vi "InvFourierTransform.vi"(2 "Complex matrix":cdb[][](array[numeric]) format="%.2f", 3 "Image In":T1 {"Dialogs" format="%.0b"}) -> (1 "Image Out":T1 {"Dialogs" format="%.0b"})   [LabVIEW 2024]
doc: "This VI calculates the inverse DFT (or FFT) of the complex matrix and returns the resulting real the image. It only works on greyscale images."
uses:
  <userlib>/ImageProcessing/QTLIB_2595_LV86/QT_Image.ctl
panel:
  # "This VI calculates the inverse DFT (or FFT) of the complex matrix and returns the resulting real the image.  It only works on greyscale images."
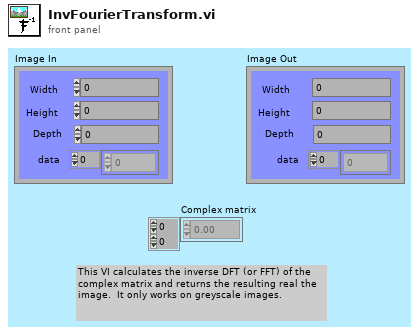
[diagram p1: front panel]
types:
  T1 = typedef "QT_Image.ctl" = cluster{"Width":i32, "Height":i32, "Depth":i32, "data":u8[], "Compressed data":u8[], "Color table":u32[], "Duration":i32, "Options":i32, "Timestamp":i32, "ID":i32, "Reserved":i32, "Dialogs":u32}
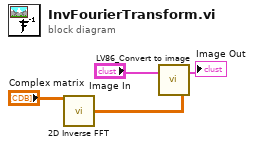
[diagram p0: block diagram]
diagram:
  n1 = call <userlib>:"2D Inverse FFT.vi"("X"="Complex matrix") -> ("FFT {X}"=w1:dbl[][])
  n2 = call <userlib>:"LV86_Convert to image.vi"("Intensity Graph"=w1, "Image In"="Image In") -> ("Image Out"=→"Image Out":T1)  [unwired: 1 in]
